vi "protocol.vi"(0 "Data in":T1={"Report.lvclass"=refnum, "test"="", "Initial State"=enum."Initialize", "test ID"=0, "parameter"=[]}, 11 "error in (no error)":errorcluster) -> (4 "Data out":T1={"Report.lvclass"=refnum, "test"="", "Initial State"=enum."Initialize", "test ID"=0, "parameter"=[]}, 15 "error out":errorcluster)   [LabVIEW 2013]
uses:
  classes/Test/Test.lvclass
  classes/Report/Report.lvclass
  Main/controls/Data.ctl
  Main/controls/State.ctl
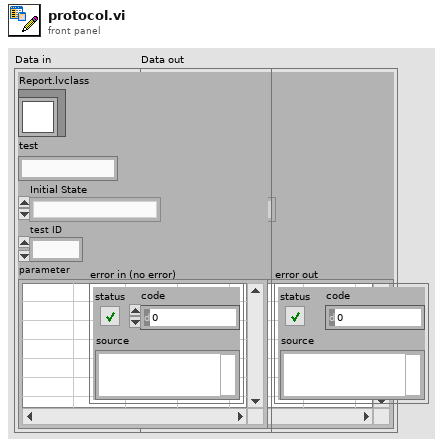
[diagram p1: front panel]
types:
  T1 = typedef "Data.ctl" = cluster{"Report.lvclass":refnum<class "Report.lvclass">, "test":string, "Initial State":T2, "test ID":i32, "parameter":string[][]}
  T2 = typedef "State.ctl" = enum16{"enter Report Parameters", "new Test", "Protokoll", "read Tree", "update Tree", "Fehler", "Initialize", "Störaussendung", "Burst", "ESD", "Surge", "Spannungseinbruch", "HF-Felder", "Wait for Event", "Exit"}
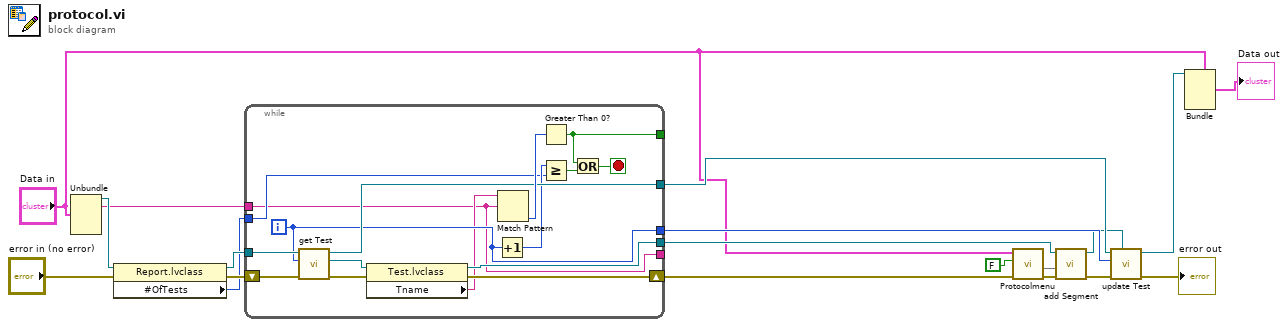
[diagram p0: block diagram]
diagram:
  n1 = Unbundle("Data in") -> ("Report.lvclass"=w21:refnum<class "Report.lvclass">, "test"=w8:string)  [unwired: 3 out]
  n2 = property class="Report.lvclass"(reference=w21, error in="error in (no error)") -> (reference out=w20:refnum<class "Report.lvclass">, error out=w19:errorcluster, "#OfTests"=w18:u32)
  n3 = while {
    tunnel: w20 -> [w37]
    shift-right: [w30] -> w13
    shift-left: w19 -> [w36]
    tunnel: w18 -> [w24]
    tunnel: [w29] -> w15
    tunnel: [w28] -> w14
    tunnel: [w27] -> w11
    tunnel: [w25] -> w12
    tunnel: w8 -> [w22]
    tunnel: [w22] -> w7
    i -> [w25]
    stop <- w32 stop-if-true
    n4 = call-dynamic "get Test.vi"("error in (no error)"=w36, "index"=w25, "Report (Eingang)"=w37) -> ("error out"=w34:errorcluster, "Test.lvclass"=w35:refnum<class "Test.lvclass">, "Report (Ausgang)"=w28:refnum<class "Report.lvclass">)  [unwired: 6 in]
    n5 = property class="Test.lvclass"(reference=w35, error in=w34) -> (reference out=w29:refnum<class "Test.lvclass">, error out=w30:errorcluster, "Tname"=w23:string)
    n6 = Increment(x=w25) -> (x+1=w26:i32)
    n7 = Match Pattern(string=w23, regular expression=w22) -> (offset past match=w33:i32)  [unwired: 1 in, 3 out]
    n8 = Greater Than 0?(x=w33) -> (x > 0?=w27:bool)
    n9 = Greater Or Equal?(x=w26, y=w24) -> (x >= y?=w31:bool)
    n10 = Or(x=w27, y=w31) -> (x .or. y?=w32:bool)
  }
  n11 = call "Protocolmenu.vi"("error in (no error)"=w13, "Parameter"=FALSE ("setup"), "Data"="Data in") -> ("error out"=w3:errorcluster, 1:w2)  [unwired: 4 in, 1 out]
  n12 = call-dynamic "add Segment.vi"("error in (no error)"=w3, "Segment.lvclass"=w2, "Test Eingang"=w15) -> ("error out"=w5:errorcluster, "Test Ausgang"=w4:refnum<class "Test.lvclass">)  [unwired: 7 in]
  n13 = call-dynamic "update Test.vi"("Test.lvclass"=w4, "error in (no error)"=w5, "index"=w12, "Report in"=w14) -> ("error out"=→"error out":errorcluster, "Report out"=w9:refnum<class "Report.lvclass">)  [unwired: 6 in]
  n14 = Bundle(cluster="Data in", "Report.lvclass"=w9) -> (→"Data out":T1)  [unwired: 4 in]
